vi "Get Wash Option.vi"(8 "Error In":errorcluster, 10 "Wash Options":T1) -> (0 "Error Out":errorcluster, 2 "Option Name":string[](array[string]))   [LabVIEW 2015, in "User Interface.lvlib" / "User Interface.lvclass"]
uses:
  User Interface.lvclass
  Controls/Wash Options.ctl
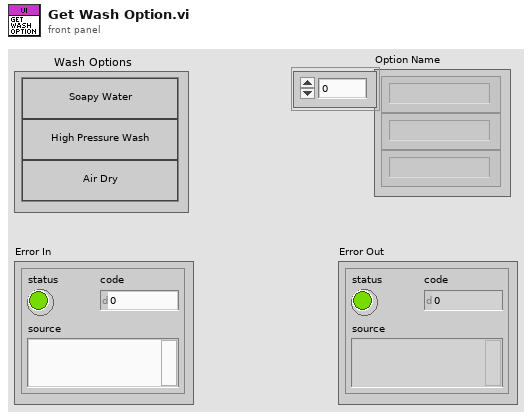
[diagram p1: front panel]
types:
  T1 = typedef "Wash Options.ctl" = cluster{"Soapy Water":bool, "High Pressure Wash":bool, "Air Dry":bool}
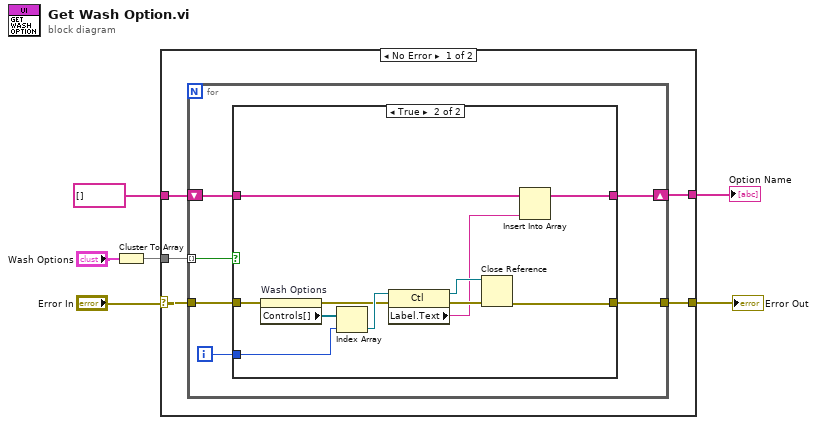
[diagram p0: block diagram]
diagram:
  n1 = Cluster To Array(cluster="Wash Options") -> (array=w4:bool[])
  n2 = case shown="No Error" "Error In" {
    selector: "Error In" -> [w10 w32]
    tunnel: w4 -> [w11 _]
    tunnel: [w9 w32] -> w3
    tunnel: string[] [] ("Option Name") -> [w8 w31]
    tunnel: [w7 w31] -> w1
    frame No Error {
      n3 = for {
        tunnel: w11 -> [w17] mode=indexing
        tunnel: w10 -> [w16]
        tunnel: [w15] -> w9
        shift-right: [w13] -> w7
        shift-left: w8 -> [w14]
        i -> [w12]
        n4 = case shown="True" w17 {
          tunnel: w16 -> [w19 w30]
          tunnel: [w19 w20] -> w15
          tunnel: w14 -> [w18 w29]
          tunnel: [w18 w28] -> w13
          tunnel: w12 -> [_ w26]
          frame False {
          }
          frame True {
            n5 = property on="Wash Options" class="Clust (strict)"(error in=w30) -> (error out=w24:errorcluster, "Controls[]"=w27:refnum<vi>[])  [unwired: 1 in, 1 out]
            n6 = Index Array(array=w27, index=w26) -> (element=w25:refnum<vi>)
            n7 = property class="Ctl"(reference=w25, error in=w24) -> (reference out=w22:refnum<vi>, error out=w23:errorcluster, "Label.Text"=w21:string)
            n8 = Close Reference(reference=w22, error in (no error)=w23) -> (error out=w20:errorcluster)
            n9 = Insert Into Array(array=w29, new element=w21) -> (w28:string[])  [unwired: 1 in]
          }
        }
      }
    }
    frame Error {
    }
  }
  "Error Out" <- w3
  "Option Name" <- w1
